vi "WriteParent.vi"(8 "error in":errorcluster, 10 "parent":T1, 11 "node in":refnum<class "NISE_CEF_Node.lvclass">) -> (0 "error out":errorcluster, 3 "node out":refnum<class "NISE_CEF_Node.lvclass">)   [LabVIEW 2013, in "NISE_CEF_Node.lvclass"]
uses:
  NISE_CEF_Node.lvclass
  NodeRef.ctl
  NISE_CEF_Node.lvclass/NISE_CEF_Node.ctl
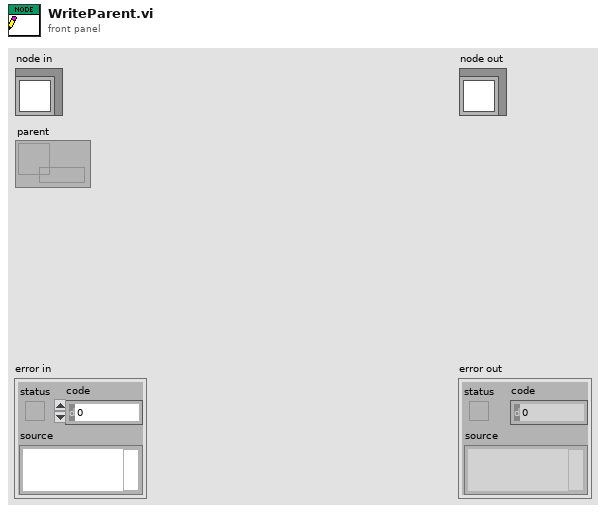
[diagram p1: front panel]
types:
  T1 = typedef "NISE_CEF_Node.lvclass/NodeRef.ctl" = refnum<data-value>
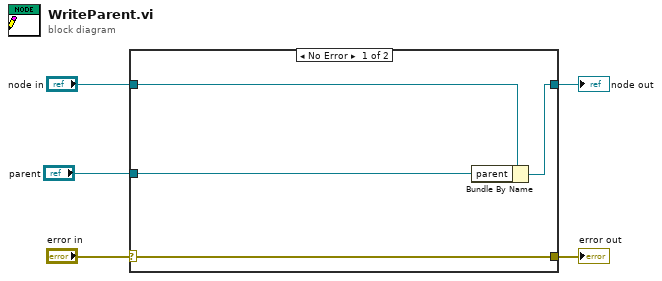
[diagram p0: block diagram]
diagram:
  n1 = case shown="No Error" "error in" {
    selector: "error in" -> [w9 w10]
    tunnel: [w9 w10] -> w4
    tunnel: [w7 w11] -> w2
    tunnel: "node in" -> [w8 w11]
    tunnel: "parent" -> [w6 _]
    frame No Error {
      n2 = Bundle By Name(cluster=w8, "parent"=w6) -> (w7:refnum<class "NISE_CEF_Node.lvclass">)
    }
    frame Error {
    }
  }
  "error out" <- w4
  "node out" <- w2
